vi "CLD 1 Elapsed Time Express Front Panel - Solution.vi"() -> ()   [LabVIEW 2020]
doc: "LabVIEW CLD 1 Exercise"
panel:
  out "error out":errorcluster
  in  "error in":errorcluster
  out "Elapsed Time":string
  out "Time has Elapsed":bool
  in  "Auto Reset":bool=TRUE
  in  "Reset Button":bool
  in  "Stop VI":bool
  in  "Time Target (s)":dbl
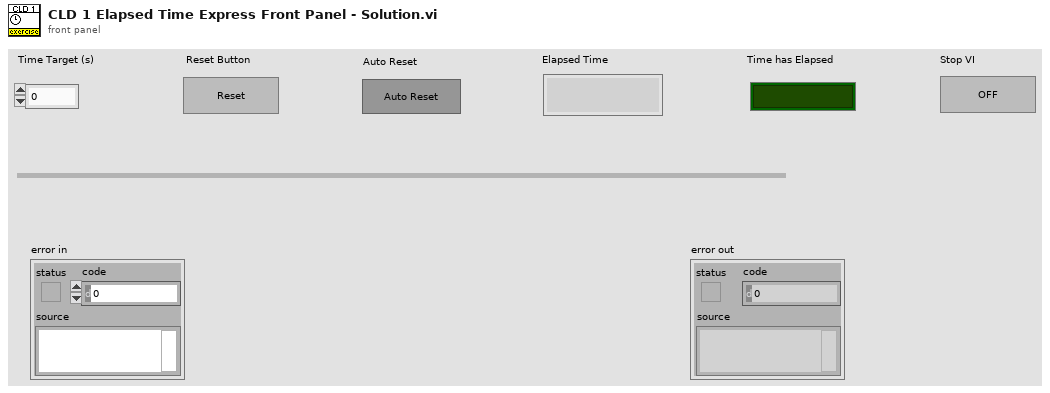
[diagram p1: front panel]
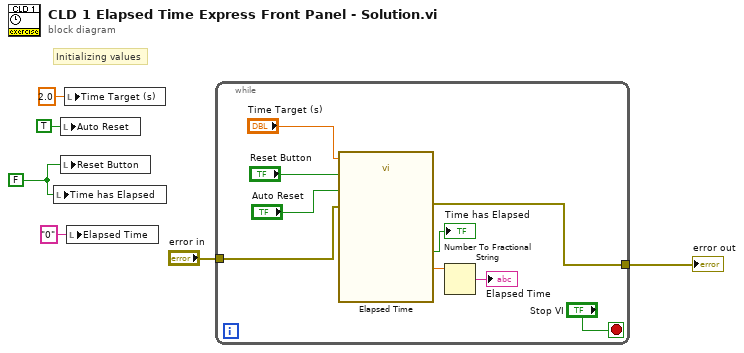
[diagram p0: block diagram]
diagram:
  w2 = FALSE ("Time has Elapsed")
  # "Initializing values"
  n1 = local write "Time has Elapsed"(w2) -> ()
  n2 = local write "Auto Reset"(TRUE ("Auto Reset")) -> ()
  n3 = local write "Reset Button"(w2) -> ()
  n4 = local write "Time Target (s)"(2.0 ("Time Target (s)")) -> ()
  n5 = local write "Elapsed Time"("0" ("Elapsed Time")) -> ()
  n6 = while {
    tunnel: "error in" -> [w8]
    tunnel: [w7] -> w5
    stop <- "Stop VI" stop-if-true
    n7 = call "Elapsed Time"("Time Target (s)"="Time Target (s)", "Reset"="Reset Button", "Auto Reset"="Auto Reset", "error in (no error)"=w8) -> ("Elapsed Time (s)"=w14:dbl, "Time has Elapsed"=→"Time has Elapsed":bool, "error out"=w7:errorcluster)  [unwired: 8 in, 5 out]
    n8 = Number To Fractional String(number=w14) -> (F-format string=→"Elapsed Time":string)  [unwired: 3 in]
  }
  "error out" <- w5
